vi "Write Sample.vi"(0 "TDMS In":refnum<k34>, 5 "InputVector":sgl[](array[numeric]), 7 "OutputVector":sgl[](array[numeric]), 11 "Error In":errorcluster) -> (4 "TDMS Out":refnum<k34>, 15 "Error Out":errorcluster)   [LabVIEW 2015, in "Teaching File.lvlib"]
doc: "Write a teaching sample into the TDMS file. \n\nThe group names used will be <b>Input_Data</b> and <b>Output_Data</b>. Channels will correspond to the index of IO in the teaching sample. If the group or the channels do not exist in TDMS, they will be created.\n\nIf the lengths of the wired samples are not matching the samples already in the file, return error 7123."
uses:
  Teaching File.lvlib
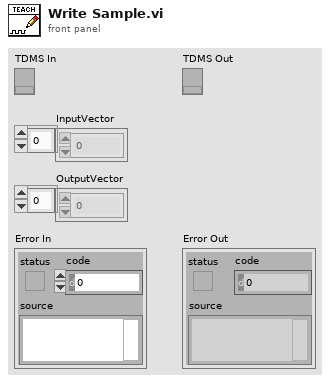
[diagram p1: front panel]
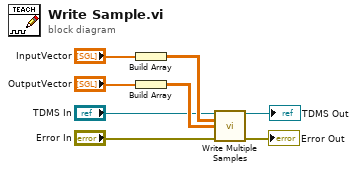
[diagram p0: block diagram]
diagram:
  n1 = Build Array("InputVector") -> (w5:sgl[][])
  n2 = Build Array("OutputVector") -> (w4:sgl[][])
  n3 = call "Write Multiple Samples.vi"("TDMS In"="TDMS In", "Input Vector"=w5, "Output Vector"=w4, "Error In"="Error In") -> ("TDMS Out"=→"TDMS Out":refnum<k34>, "Error Out"=→"Error Out":errorcluster)  [unwired: 10 in]
